vi "GetPositionUm.vi"(8 "error in (no error)":errorcluster, 10 "Stage Label":string, 11 "Stage in":refnum<class "Stage.lvclass">) -> (0 "error out":errorcluster, 2 "Stage Position":dbl, 3 "Stage out":refnum<class "Stage.lvclass">)   [LabVIEW 2020, in "Stage.lvlib" / "Stage.lvclass"]
uses:
  Stage.lvclass
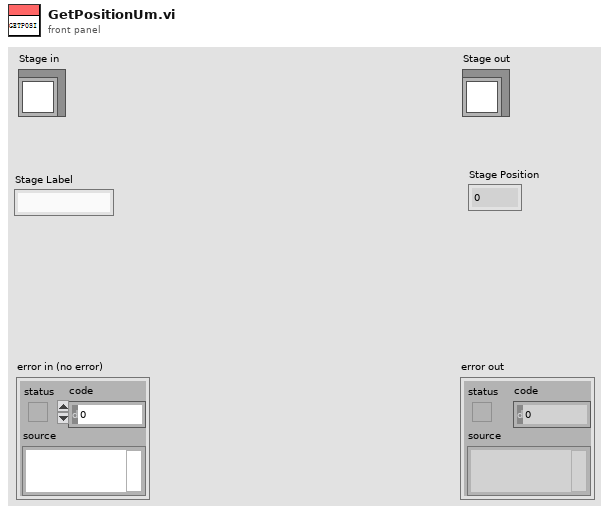
[diagram p1: front panel]
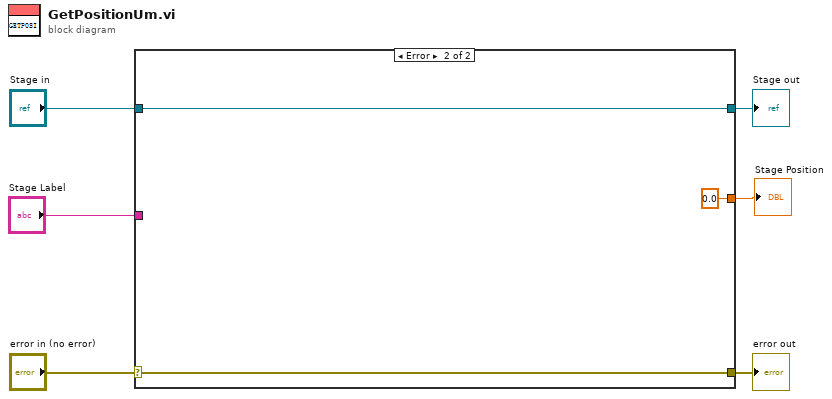
[diagram p0: block diagram]
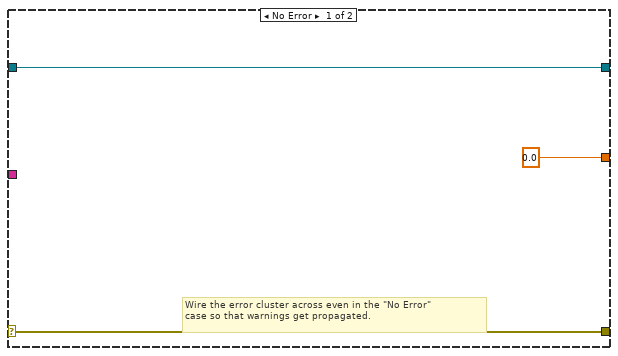
[diagram p2: hidden frame]
diagram:
  n1 = case shown="Error" "error in (no error)" {
    selector: "error in (no error)" -> [w8 w12]
    tunnel: [w8 w12] -> w5
    tunnel: [w9 w11] -> w3
    tunnel: "Stage in" -> [w9 w11]
    tunnel: "Stage Label" -> [_ _]
    tunnel: [0.0 0.0] -> w1
    frame No Error {
      # "Wire the error cluster across even in the \"No Error\"\ncase so that warnings get propagated."
    }
    frame Error {
    }
  }
  "error out" <- w5
  "Stage out" <- w3
  "Stage Position" <- w1
